vi "SettingPanelKEITHLEY2182andKEITHLEY6222.vi"(11 "KEITHLEY2182andKEITHLEY6222_In":refnum<vi>) -> (3 "KEITHLEY2182andKEITHLEY6222_out":refnum<vi>)   [LabVIEW 2013]
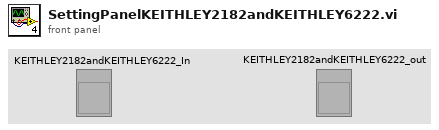
[diagram p1: front panel]
types:
  T1 = enum8{"Enabled", "Disabled", "Disabled and Grayed Out"}
  T2 = typedef "Keithly user program.lvlib/KE2182 -- Params.ctl" = cluster{"Auto Range?":bool, "Man / Selected\n       Range":enum16{"10mV", "100mV", "1V", "10V", "100V"}, "Enable Digital\n       Filter?":bool, "Filter Type":enum16{"Movin", "Repeat"}, "Filter Count":u32, "      Filter\nWindow (%)":dbl, "Enable Analog\n       Filter?":bool, "NPLCs":u32}
  T3 = typedef "Keithly user program.lvlib/KE622x -- Current Range.ctl" = cluster{"Auto Range?":bool, "Man / Selected\n        Range":enum16{"2nA", "20nA", "200nA", "2uA", "20uA", "200uA", "2mA", "20mA", "100mA"}}
  T4 = typedef "Keithly user program.lvlib/KE622x -- Current Level.ctl" = dbl
  T5 = typedef "Keithly user program.lvlib/KE622x -- Voltage Limit.ctl" = dbl
  T6 = typedef "Keithly user program.lvlib/KE6221 -- Output Response.ctl" = enum16{"Fast", "Slow"}
  T7 = cluster{"KEITHLEY ON/OFF":bool, "VISA KEITHLEY resource name":refnum<visa-resource-name>, "2182 -A Params":T2, "KEITHLEY CURRENT ON/OFF":bool, "6221 Params":cluster{"Current Range":T3, "Current Level (A)":T4, "Voltage Limit (V)":T5, "KE6221 Output Response":T6, "Analog Filter State":enum16{"Off", "On"}}, "Step Mode\nParams":bool, "Step Mode":cluster{"Front Point (A)":T4, "Start Point (A)":T4, "Back Point (A)":T4, "Step(A)":T4, "Time step (ms)":dbl, "N cycle":dbl, "Sweeping":enum16{"Off Sweeping", "On Sweeping"}, "Go to":enum16{"Star Point", "Back Point"}}}
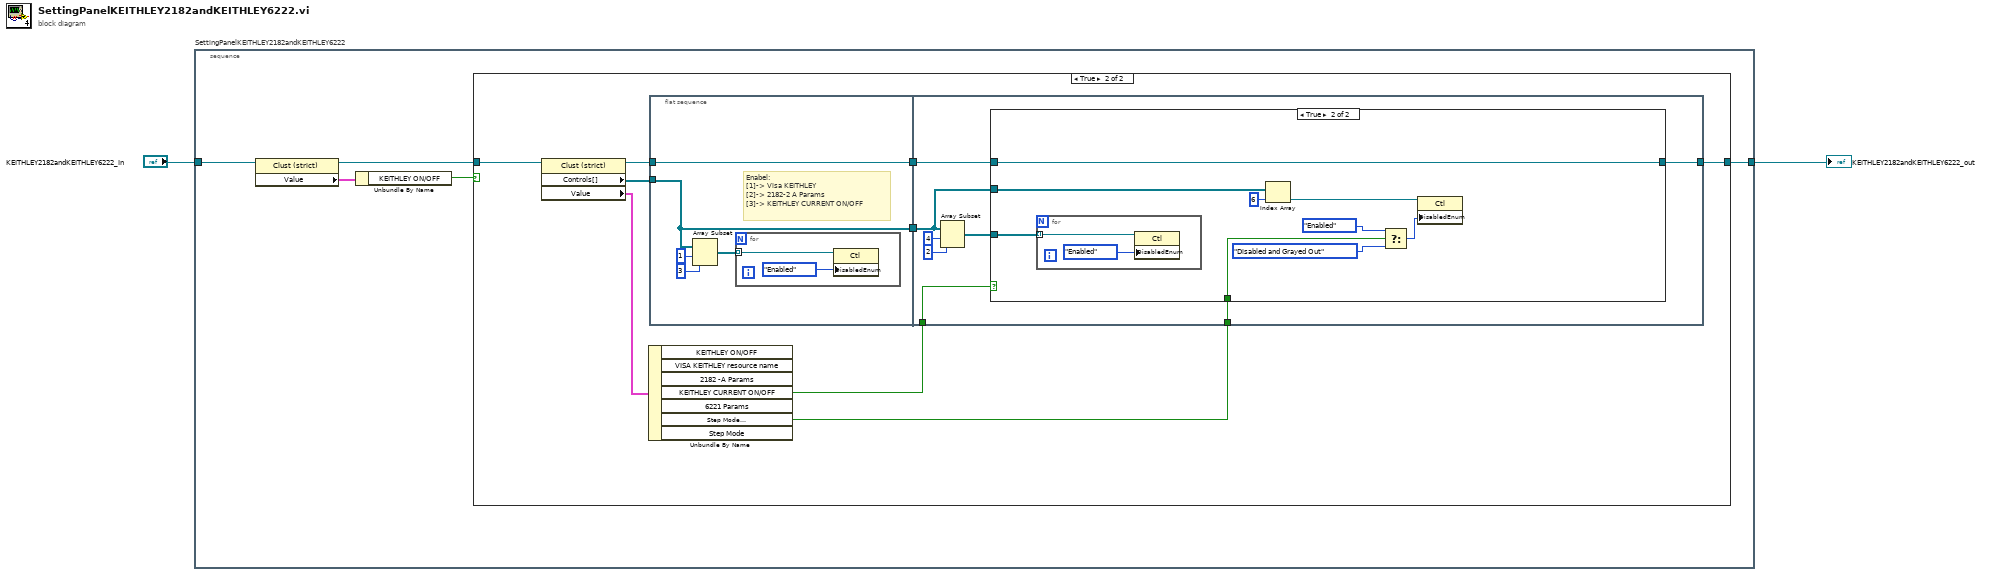
[diagram p0: block diagram]
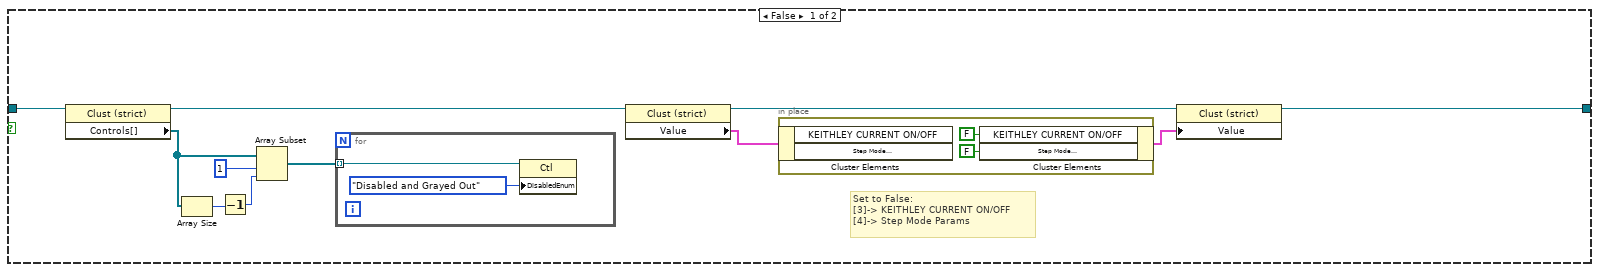
[diagram p2: hidden frame]
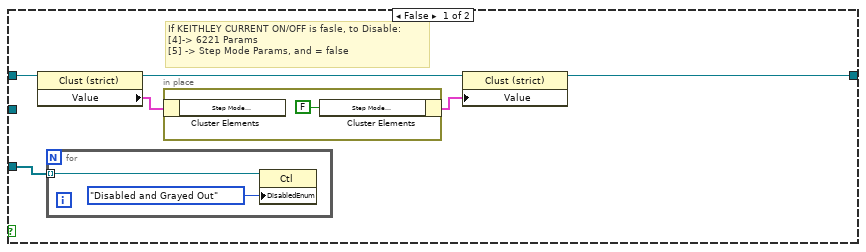
[diagram p3: hidden frame]
diagram:
  n1 = stacked-sequence "SettingPanelKEITHLEY2182andKEITHLEY6222" {
    tunnel: "KEITHLEY2182andKEITHLEY6222_In" -> [w7]
    tunnel: [w4] -> w2
    frame #0 {
      n2 = property class="Clust (strict)"(reference=w7) -> (reference out=w5:refnum<vi>, "Value"=w6:T7)  [unwired: 1 in, 1 out]
      n3 = Unbundle By Name(w6) -> ("KEITHLEY ON/OFF"=w3:bool)
      n4 = case shown="True" w3 {
        tunnel: w5 -> [w18 w31]
        tunnel: [w12 w24] -> w4
        frame False {
          # "Set to False:\n[3]-> KEITHLEY CURRENT ON/OFF\n[4]-> Step Mode Params"
          n5 = property class="Clust (strict)"(reference=w18) -> (reference out=w11:refnum<vi>, "Controls[]"=w16:refnum<vi>[])  [unwired: 1 in, 1 out]
          n6 = Array Size(array=w16) -> (size(s)=w15:i32)
          n7 = Decrement(x=w15) -> (x-1=w14:i32)
          n8 = Array Subset(array=w16, index=1, length=w14) -> (w13:refnum<vi>[])
          n9 = for {
            tunnel: w13 -> [w22] mode=indexing
            n10 = property class="Ctl"(reference=w22, "DisabledEnum"=T1."Disabled and Grayed Out" ("Disabled")) -> ()  [unwired: 1 in, 2 out]
          }
          n11 = property class="Clust (strict)"(reference=w11) -> (reference out=w10:refnum<vi>, "Value"=w9:T7)  [unwired: 1 in, 1 out]
          n12 = in-place {
            n13 = in-place-cluster #1(w9) -> ()  [unwired: 2 out]
            n14 = in-place-cluster #1("KEITHLEY CURRENT ON/OFF"=FALSE, "Step Mode\nParams"=FALSE ("Step Mode\nParams")) -> (w8:T7)
          }
          n15 = property class="Clust (strict)"(reference=w10, "Value"=w8) -> (reference out=w12:refnum<vi>)  [unwired: 1 in, 1 out]
        }
        frame True {
          n16 = property class="Clust (strict)"(reference=w31) -> (reference out=w26:refnum<vi>, "Controls[]"=w29:refnum<vi>[], "Value"=w30:T7)  [unwired: 1 in, 1 out]
          n17 = Unbundle By Name(w30) -> ("KEITHLEY CURRENT ON/OFF"=w27:bool, "Step Mode\nParams"=w23:bool)  [unwired: 5 out]
          n18 = flat-sequence {
            tunnel: w29 -> [w33]
            tunnel: [w33] -> w28
            tunnel: w26 -> [w32]
            tunnel: [w32] -> w25
            tunnel: w28 -> [w40]
            tunnel: w27 -> [w44]
            tunnel: w25 -> [w42]
            tunnel: [w41] -> w24
            tunnel: w23 -> [w39]
            frame #0 {
              # "Enabel:\n[1]-> Visa KEITHLEY\n[2]-> 2182-2 A Params\n[3]-> KEITHLEY CURRENT ON/OFF"
              n19 = Array Subset(array=w33, index=1, length=3) -> (w34:refnum<vi>[])
              n20 = for {
                tunnel: w34 -> [w38] mode=indexing
                n21 = property class="Ctl"(reference=w38, "DisabledEnum"=T1."Enabled" ("Disabled")) -> ()  [unwired: 1 in, 2 out]
              }
            }
            frame #1 {
              n22 = Array Subset(array=w40, index=4, length=2) -> (w43:refnum<vi>[])
              n23 = case shown="True" w44 {
                tunnel: w43 -> [w52 w64]
                tunnel: w42 -> [w51 w63]
                tunnel: [w47 w63] -> w41
                tunnel: w40 -> [_ w62]
                tunnel: w39 -> [_ w59]
                frame False {
                  # "If KEITHLEY CURRENT ON/OFF is fasle, to Disable:\n[4]-> 6221 Params\n[5] -> Step Mode Params, and = false"
                  n24 = property class="Clust (strict)"(reference=w51) -> (reference out=w50:refnum<vi>, "Value"=w49:T7)  [unwired: 1 in, 1 out]
                  n25 = for {
                    tunnel: w52 -> [w55] mode=indexing
                    n26 = property class="Ctl"(reference=w55, "DisabledEnum"=T1."Disabled and Grayed Out" ("Disabled")) -> ()  [unwired: 1 in, 2 out]
                  }
                  n27 = in-place {
                    n28 = in-place-cluster #2(w49) -> ()  [unwired: 1 out]
                    n29 = in-place-cluster #2("Step Mode\nParams"=FALSE ("Step Mode\nParams")) -> (w48:T7)
                  }
                  n30 = property class="Clust (strict)"(reference=w50, "Value"=w48) -> (reference out=w47:refnum<vi>)  [unwired: 1 in, 1 out]
                }
                frame True {
                  n31 = for {
                    tunnel: w64 -> [w66] mode=indexing
                    n32 = property class="Ctl"(reference=w66, "DisabledEnum"=T1."Enabled" ("Disabled")) -> ()  [unwired: 1 in, 2 out]
                  }
                  n33 = Index Array(array=w62, index=6) -> (element=w60:refnum<vi>)
                  n34 = Select(t=T1."Enabled" ("Disabled"), s=w59, f=T1."Disabled and Grayed Out" ("Disabled")) -> (s? t:f=w56:T1)
                  n35 = property class="Ctl"(reference=w60, "DisabledEnum"=w56) -> ()  [unwired: 1 in, 2 out]
                }
              }
            }
          }
        }
      }
    }
  }
  "KEITHLEY2182andKEITHLEY6222_out" <- w2
